vi "Search and Replace Pattern regex2.vi"(6 "offset (0)":i32, 7 "replace all? (F)":bool, 8 "error in":errorcluster, 9 "replace string (\"\")":string, 10 "regular expression (\"\")":string, 11 "string":string) -> (0 "error out":errorcluster, 1 "offset past match":i32, 3 "result string":string)   [LabVIEW 2019]
doc: "Searches <B>string</B> for substrings that match <B>regular expression</B> and replaces those substrings with <B>replace string</B>. A regular expression requires a specific combination of characters for pattern matching. For more information about special characters in regular expressions, refer to the <B>regular expression</B> input description in the detailed help.\nThis version uses Match Regular Expression instead of Match Pattern to support full regular expression syntax"
uses:
  <vilib>/regexp/Match Regular Expression.xnode
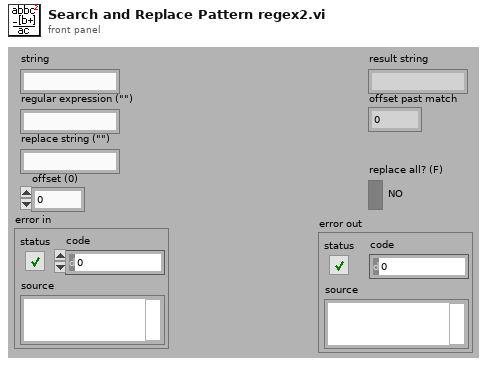
[diagram p1: front panel]
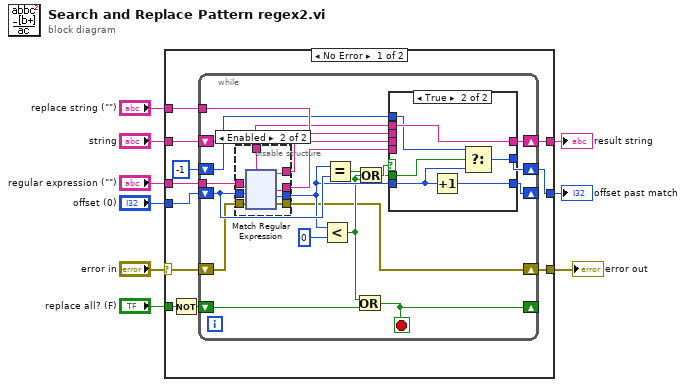
[diagram p0: block diagram]
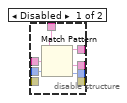
[diagram p2: hidden frame]
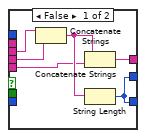
[diagram p3: hidden frame]
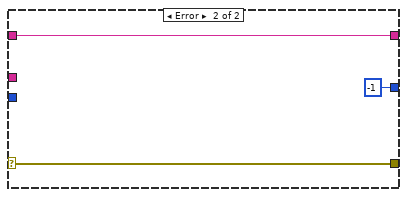
[diagram p4: hidden frame]
diagram:
  n1 = case shown="No Error" "error in" {
    selector: "error in" -> [w10 w180]
    tunnel: "replace all? (F)" -> [w20 _]
    tunnel: "string" -> [w19 w181]
    tunnel: "replace string (\"\")" -> [w18 _]
    tunnel: "regular expression (\"\")" -> [w17 _]
    tunnel: [w15 w181] -> w5
    tunnel: "offset (0)" -> [w14 _]
    tunnel: [w13 -1] -> w3
    tunnel: [w11 w180] -> w2
    frame No Error {
      n2 = Not(x=w20) -> (.not. x?=w16:bool)
      n3 = while {
        shift-right: [w33] -> _
        shift-left: w16 -> [w34]
        shift-right: [w31] -> _
        shift-left: w14 -> [w27]
        shift-right: [w35] -> w15
        shift-left: w19 -> [w32]
        tunnel: w17 -> [w39]
        tunnel: w18 -> [w36]
        shift-right: [w25] -> w13
        shift-left: -1 -> [w24]
        shift-right: [w21] -> w11
        shift-left: w10 -> [w22]
        stop <- w33 stop-if-true
        n4 = disable-structure shown="Enabled" {
          disable-tunnel: w39 -> [w45 w52]
          disable-tunnel: [w44 w48] -> w38
          disable-tunnel: [w43 w47] -> w37
          disable-tunnel: w32 -> [w42 w53]
          disable-tunnel: w27 -> [w41 w51]
          disable-tunnel: [w40 w46] -> w26
          disable-tunnel: w22 -> [_ w50]
          disable-tunnel: [_ w49] -> w21
          frame Disabled {
            n5 = Match Pattern(string=w42, regular expression=w45, offset (0)=w41) -> (before substring=w44:string, after substring=w43:string, offset past match=w40:i32)  [unwired: 1 out]
          }
          frame Enabled {
            n6 = xnode "Match Regular Expression"("input string"=w53, "regular expression"=w52, "offset (0)"=w51, "error in"=w50) -> ("before match"=w48:string, "after match"=w47:string, "offset past match"=w46:i32, "error out"=w49:errorcluster)  [unwired: 2 in, 1 out]
          }
        }
        n7 = Less?(x=w26, y=0) -> (x < y?=w23:bool)
        n8 = Equal?(x=w26, y=w27) -> (x = y?=w28:bool)
        n9 = Or(x=w23, y=w34) -> (x .or. y?=w33:bool)
        n10 = Or(x=w28, y=w23) -> (x .or. y?=w29:bool)
        n11 = case shown="True" w29 {
          tunnel: w38 -> [w172 _]
          tunnel: w37 -> [w169 _]
          tunnel: w36 -> [w171 _]
          tunnel: [w173 w179] -> w35
          tunnel: w32 -> [_ w179]
          tunnel: [w168 w178] -> w31
          tunnel: w26 -> [_ w175]
          tunnel: [w168 w174] -> w25
          tunnel: w24 -> [_ w176]
          tunnel: w23 -> [_ w177]
          frame False {
            n12 = Concatenate Strings(w172, w171) -> (w170:string)
            n13 = Concatenate Strings(w170, w169) -> (w173:string)
            n14 = String Length(string=w170) -> (length=w168:i32)
          }
          frame True {
            n15 = Increment(x=w175) -> (x+1=w178:i32)
            n16 = Select(t=w176, s=w177, f=w175) -> (s? t:f=w174:i32)
          }
        }
      }
    }
    frame Error {
    }
  }
  "result string" <- w5
  "offset past match" <- w3
  "error out" <- w2
